vi "Field Draw Robot.vi"(0 "Offset":T5, 1 "picture in":picture, 3 "Draw Number":bool, 5 "Robot":refnum<class "Robot.lvclass">=refnum, 6 "Project":T1=enum."VSS", 7 "Game in":refnum<class "Game.lvclass">=refnum, 9 "Scale mm/pixel":sgl, 11 "color(black)":u32(colorbox)=16775978, 12 "Lado":enum16{"Esquerdo", "Direito"}(ring), 14 "color":enum16{"Azul", "Amarelo"}(ring), 15 "Draw Targets?":T3) -> (4 "picture out":picture)   [LabVIEW 2022 SP3]
uses:
  <vilib>/Analysis/NI_AALPro.lvlib
  <vilib>/Analysis/coordinate.llb/2D Cartesian Coordinate Rotation (Scalar).vi
  Controls/Functions Enum.ctl
  Robot_class/Robot.lvclass
  Game_class/Game.lvclass
  Enemy_class/Enemy.lvclass
  Referee_class/Referee.lvclass
  <vilib>/Utility/miscctls.llb/LVBoundsTypeDef.ctl
  DrawTargets.ctl
  Project.ctl
panel:
  in  "pen Chute 2":T2={"Width"=3, "Style"=enum."Solid"}
  in  "pen Chute":T2={"Width"=3, "Style"=enum."Solid"}
  in  "pen":T4={"Width"=1.0, "Style"=enum."Solid"}
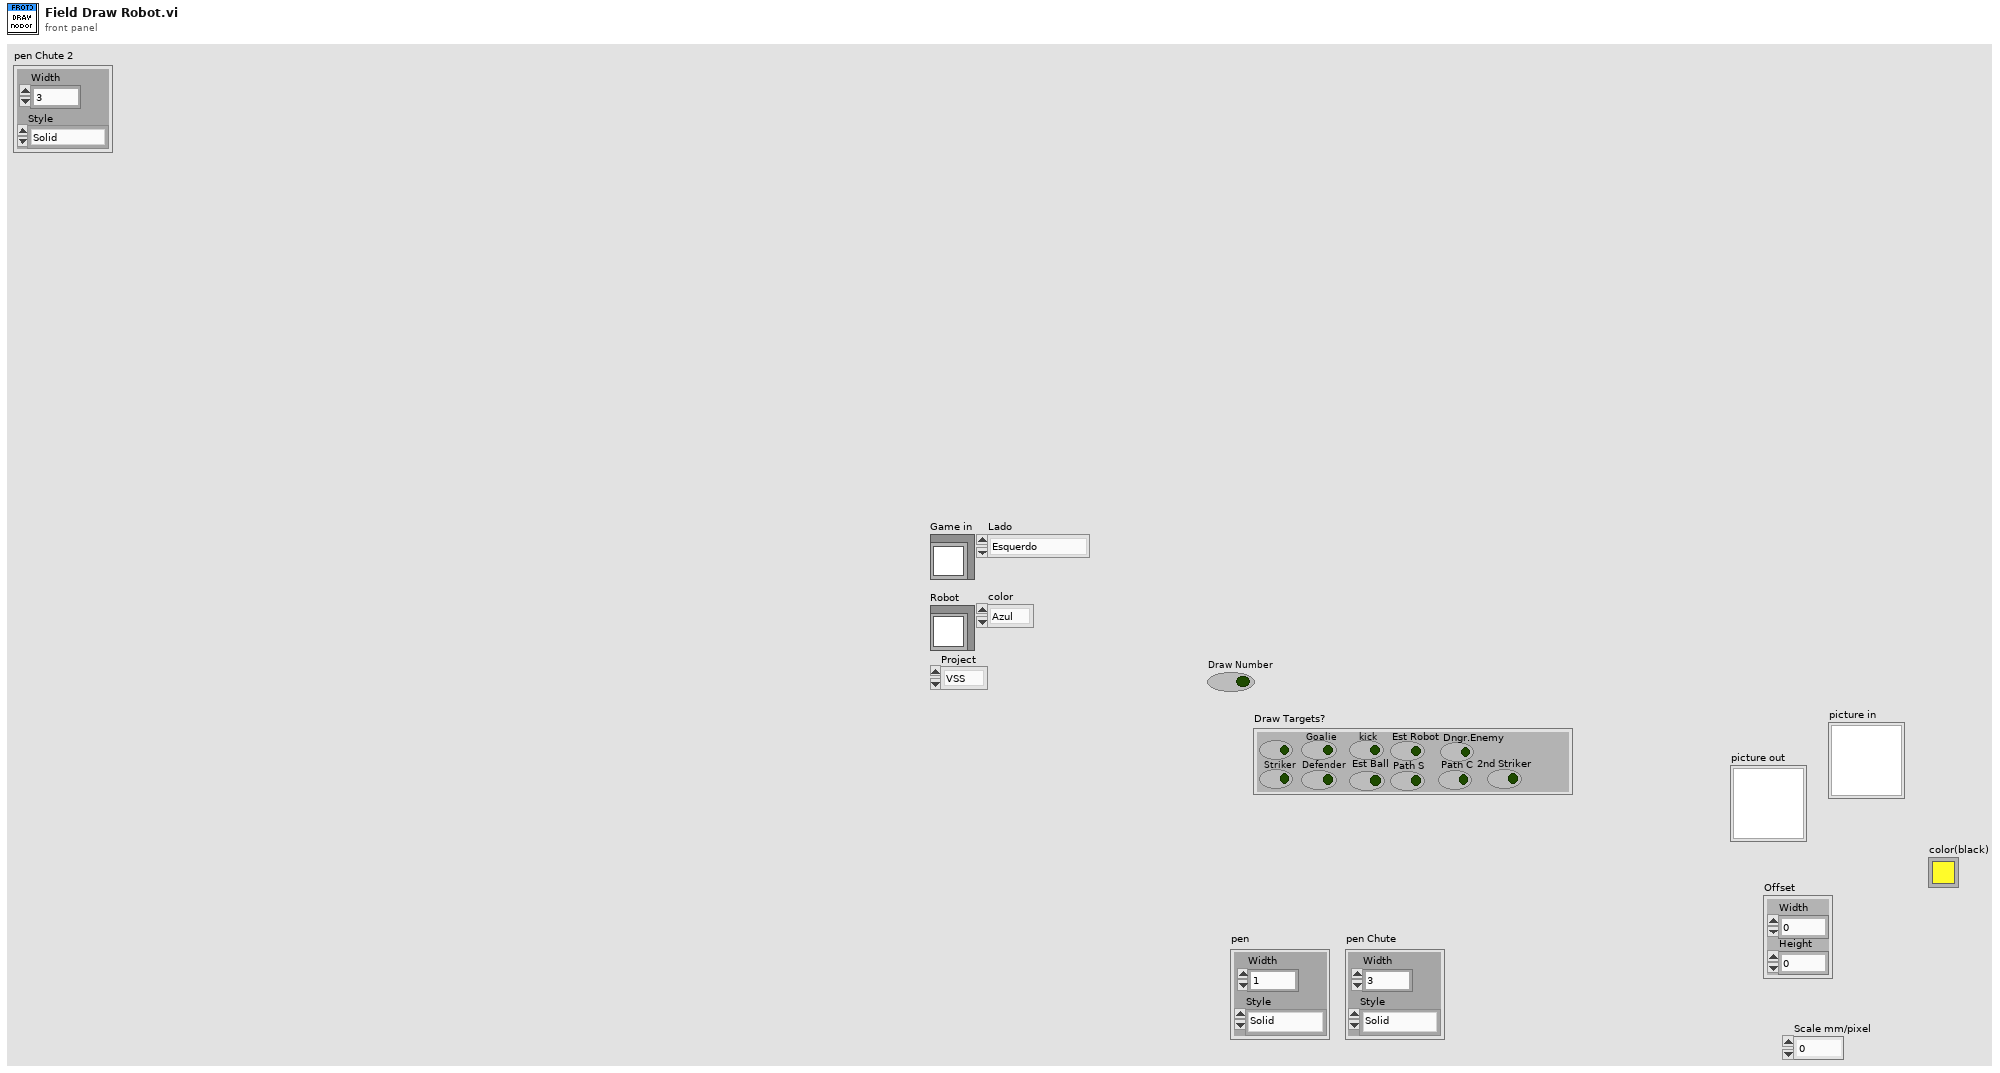
[diagram p1: front panel]
types:
  T1 = typedef "Project.ctl" = enum16{"SSL", "VSS"}
  T2 = cluster{"Width":u16, "Style":enum32{"Solid", "Dash", "Dot", "DashDot", "DashDotDot"}}
  T3 = typedef "DrawTargets.ctl" = cluster{"Attacker":bool, "Striker":bool, "Goalie":bool, "Defender":bool, "kick":bool, "Est Ball":bool, "Est Robot":bool, "Path S":bool, "Path C":bool, "Dngr.Enemy":bool, "2nd Striker":bool}
  T4 = cluster{"Width":dbl, "Style":enum32{"Solid", "Dash", "Dot", "DashDot", "DashDotDot"}}
  T5 = typedef "LVBoundsTypeDef.ctl" = cluster{"Width":u32, "Height":u32}
  T6 = typedef "Functions Enum.ctl" = enum16{"2nd Striker", "Attacker", "Goalie", "Defender", "Striker", "Goto 0", "Dummy", "Kicker", "ZigZag 0", "ZigZag 1", "ZigZag 2", "ZigZag 3", "ZigZag 4", "ZigZag 5", "ZigZag 6", "ZigZag 7", "ZigZag 8", ""}
  T7 = cluster{"horizontal":enum16{"left", "center", "right"}, "vertical":enum16{"top", "center", "bottom"}}
  T8 = typedef "dangerEnemy.ctl" = cluster{"dangerFactor":dbl, "allyRobotId":i32, "enemyRobotId":i32}
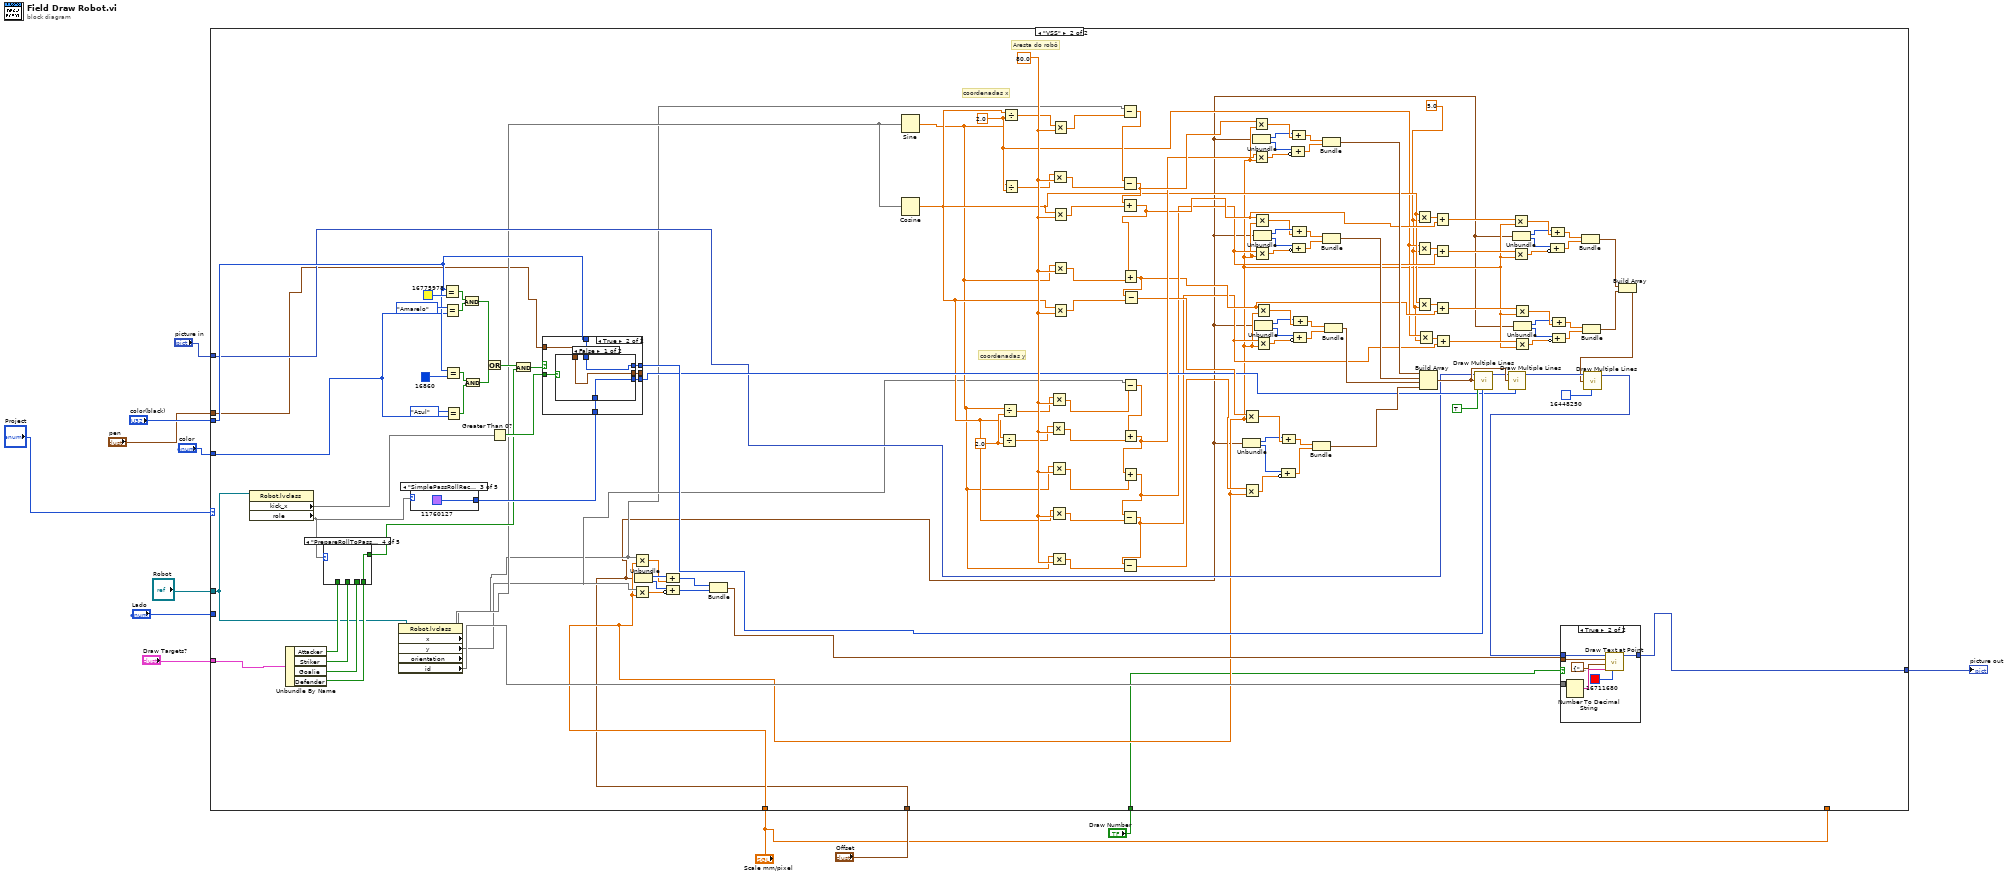
[diagram p0: block diagram]
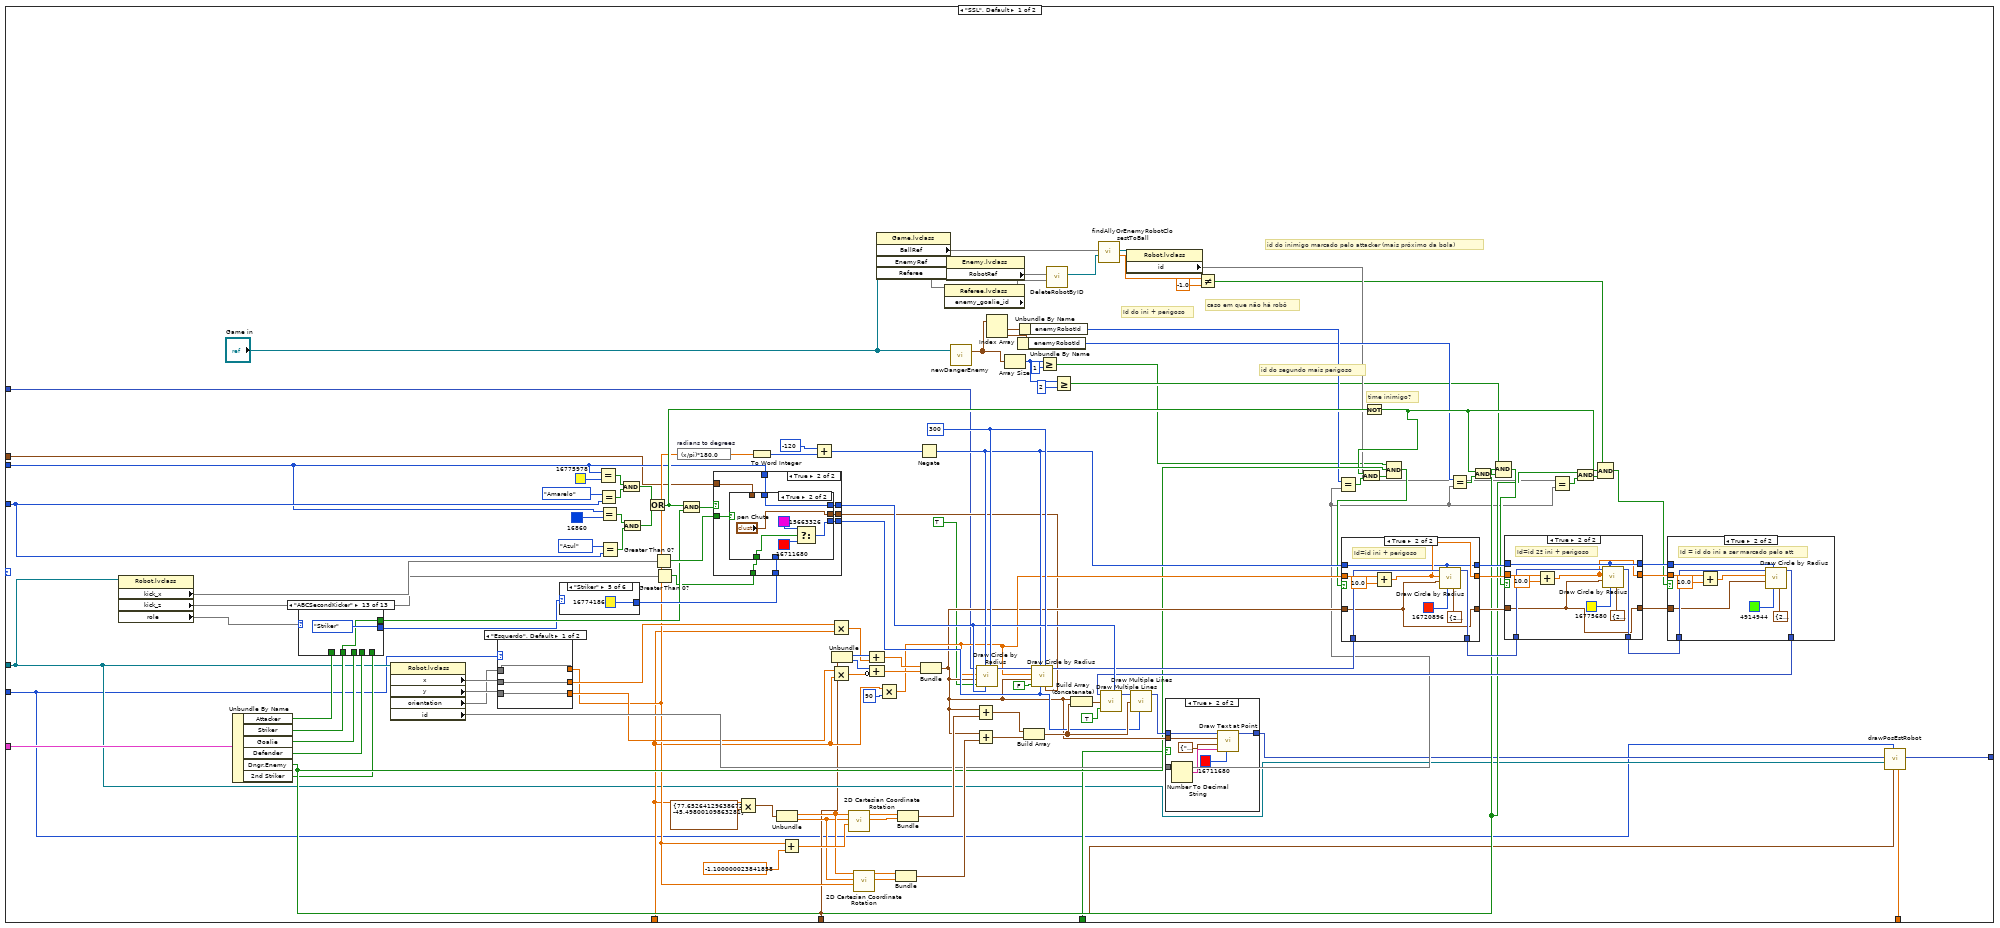
[diagram p2: hidden frame]
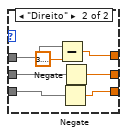
[diagram p3: hidden frame]
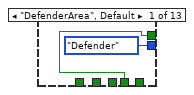
[diagram p7: hidden frame]
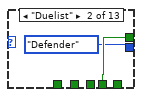
[diagram p8: hidden frame]
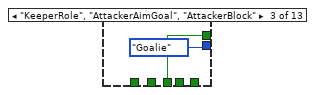
[diagram p9: hidden frame]
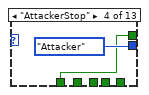
[diagram p10: hidden frame]
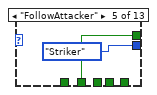
[diagram p11: hidden frame]
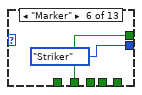
[diagram p12: hidden frame]
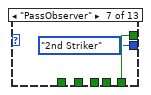
[diagram p13: hidden frame]
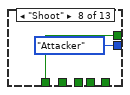
[diagram p14: hidden frame]
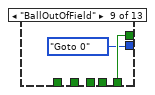
[diagram p15: hidden frame]
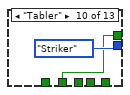
[diagram p16: hidden frame]
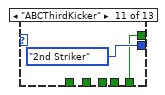
[diagram p17: hidden frame]
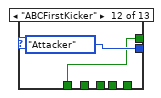
[diagram p18: hidden frame]
diagram:
  n1 = case shown="\"VSS\"" "Project" {
    tunnel: "Robot" -> [w19 w252]
    tunnel: "Draw Targets?" -> [w49 w257]
    tunnel: "color" -> [w48 w246]
    tunnel: "color(black)" -> [w47 w261]
    tunnel: [w17 w247] -> w8
    tunnel: "Draw Number" -> [w46 w248]
    tunnel: "picture in" -> [w45 w258]
    tunnel: "pen" -> [w44 w251]
    tunnel: "Offset" -> [w18 w249]
    tunnel: "Scale mm/pixel" -> [w43 w250]
    tunnel: "Lado" -> [w15 _]
    tunnel: "Scale mm/pixel" -> [w16 _]
    frame "SSL", Default {
      w129 = i16 300 ("arc size(360)")
      # "caso em que não há robô"
      # "id do inimigo marcado pelo attacker (mais próximo da bola)"
      # "id do segundo mais perigoso"
      # "time inimigo?"
      # "Id do ini + perigoso"
      n2 = property class="Robot.lvclass"(reference=w19) -> ("kick_x"=w58, "kick_z"=w14, "role"=w56)  [unwired: 1 in, 2 out]
      n3 = Unbundle By Name(w49) -> ("Attacker"=w93:bool, "Striker"=w92:bool, "Goalie"=w91:bool, "Defender"=w90:bool, "Dngr.Enemy"=w63:bool, "2nd Striker"=w60:bool)
      n4 = case shown="\"ABCSecondKicker\"" w56 {
        tunnel: [w187 w190 w192 w193 w196 w198 w200 w202 w204 w205 w207 w209 w211] -> w88
        tunnel: w90 -> [w187 w190 _ _ _ _ _ _ _ _ _ _ _]
        tunnel: w92 -> [_ _ _ _ w196 w198 _ _ _ w205 _ _ w211]
        tunnel: w93 -> [_ _ _ w193 _ _ _ w202 _ _ _ w209 _]
        tunnel: w91 -> [_ _ w192 _ _ _ _ _ _ _ _ _ _]
        tunnel: w60 -> [_ _ _ _ _ _ w200 _ w204 _ w207 _ _]
        tunnel: [Functions_Enum."Defender" ("function") Functions_Enum."Defender" ("function") Functions_Enum."Goalie" ("function") Functions_Enum."Attacker" ("function") Functions_Enum."Striker" ("function") Functions_Enum."Striker" ("function") Functions_Enum."2nd Striker" ("function") Functions_Enum."Attacker" ("function") Functions_Enum."Goto 0" ("function") Functions_Enum."Striker" ("function") Functions_Enum."2nd Striker" ("function") Functions_Enum."Attacker" ("function") Functions_Enum."Striker" ("function")] -> w57
        frame "DefenderArea", Default {
        }
        frame "Duelist" {
        }
        frame "KeeperRole", "AttackerAimGoal", "AttackerBlock" {
        }
        frame "AttackerStop" {
        }
        frame "FollowAttacker" {
        }
        frame "Marker" {
        }
        frame "PassObserver" {
        }
        frame "Shoot" {
        }
        frame "BallOutOfField" {
        }
        frame "Tabler" {
        }
        frame "ABCThirdKicker" {
        }
        frame "ABCFirstKicker" {
        }
        frame "ABCSecondKicker" {
        }
      }
      n5 = property class="Robot.lvclass"(reference=w19) -> ("x"=w55, "y"=w53, "orientation"=w51, "id"=w59)  [unwired: 1 in, 2 out]
      n6 = case shown="\"Esquerdo\", Default" w15 {
        tunnel: [w143 w150] -> w54
        tunnel: w55 -> [w143 w147]
        tunnel: [w142 w148] -> w52
        tunnel: w53 -> [w142 w149]
        tunnel: w51 -> [w141 w145]
        tunnel: [w141 w146] -> w50
        frame "Esquerdo", Default {
        }
        frame "Direito" {
          n7 = Subtract(x=w145, y=3.141592653589793) -> (x-y=w146:dbl)
          n8 = Negate(x=w149) -> (-x=w148:dbl)
          n9 = Negate(x=w147) -> (-x=w150:dbl)
        }
      }
      n10 = case shown="\"Striker\"" w57 {
        tunnel: [u32 14047743 ("color(black)") u32 16711680 ("color(black)") u32 11760127 ("color(black)") u32 4390883 ("color(black)") u32 16774186 ("color(black)") u32 197379 ("color(black)")] -> w95
        frame "Goalie" {
        }
        frame "Attacker", Default {
        }
        frame "Goto 0", "Kicker", "ZigZag 0" {
        }
        frame "Defender" {
        }
        frame "Striker" {
        }
        frame "2nd Striker" {
        }
      }
      n11 = Equal?(x=w47, y=u32 16775978 ("color(black)")) -> (x = y?=w102:bool)
      n12 = Equal?(x=enum16{"Azul", "Amarelo"}."Amarelo", y=w48) -> (x = y?=w103:bool)
      n13 = Equal?(x=w47, y=u32 16860 ("color(black)")) -> (x = y?=w99:bool)
      n14 = Equal?(x=enum16{"Azul", "Amarelo"}."Azul", y=w48) -> (x = y?=w100:bool)
      n15 = And(x=w102, y=w103) -> (x .and. y?=w97:bool)
      n16 = And(x=w99, y=w100) -> (x .and. y?=w96:bool)
      n17 = Or(x=w97, y=w96) -> (x .or. y?=w74:bool)
      n18 = Greater Than 0?(x=w58) -> (x > 0?=w94:bool)
      n19 = Greater Than 0?(x=w14) -> (x > 0?=w13:bool)
      n20 = expression code="(x/pi)*180.0" "radians to degrees"(w50) -> (w132:dbl)
      n21 = And(x=w74, y=w88) -> (x .and. y?=w89:bool)
      n22 = case shown="True" w89 {
        tunnel: [w214 w222] -> w107
        tunnel: [w214 w221] -> w106
        tunnel: w47 -> [w214 w220]
        tunnel: w95 -> [_ w219]
        tunnel: [w213 w218] -> w82
        tunnel: w94 -> [_ w217]
        tunnel: w44 -> [w213 w216]
        tunnel: w13 -> [_ w215]
        frame False {
        }
        frame True {
          n23 = case shown="True" w217 {
            tunnel: [w224 w226] -> w221
            tunnel: w220 -> [w225 w231]
            tunnel: [w225 w231] -> w222
            tunnel: w219 -> [w224 _]
            tunnel: [w223 "pen Chute"] -> w218
            tunnel: w216 -> [w223 _]
            tunnel: w215 -> [_ w229]
            frame False {
            }
            frame True {
              n24 = Select(t=u32 15663326 ("color(black)"), s=w229, f=u32 16711680 ("color(black)")) -> (s? t:f=w226:u32)
            }
          }
        }
      }
      n25 = Multiply(x=w43, y=cluster{sgl, sgl} {77.65264, -45.498} ("appended array")) -> (x*y=w113:cluster{sgl, sgl})
      n26 = To Word Integer(number=w132) -> (16bit integer=w131:i16)
      n27 = Unbundle(w113) -> (w118:sgl, w117:sgl)
      n28 = Add(x=w50, y=sgl -1.1 ("theta")) -> (x+y=w119:sgl)
      n29 = Add(x=i16 -120, y=w131) -> (x+y=w130:i16)
      n30 = Multiply(x=w54, y=w43) -> (x*y=w138:sgl)
      n31 = Multiply(x=w52, y=w43) -> (x*y=w135:sgl)
      n32 = Unbundle(w18) -> ("Width"=w139:u32, "Height"=w136:u32)
      n33 = call-poly <vilib>:"2D Cartesian Coordinate Rotation.vi"("theta"=w119, "y"=w117, "x"=w118) -> ("y out"=w121:dbl, "x out"=w122:dbl)  [unwired: 6 in, 1 out]
      n34 = call-poly <vilib>:"2D Cartesian Coordinate Rotation.vi"("theta"=w50, "y"=w117, "x"=w118) -> ("y out"=w115:dbl, "x out"=w116:dbl)  [unwired: 6 in, 1 out]
      n35 = Compound Arithmetic op=ADD(w139, w138) -> (w137:sgl)
      n36 = Compound Arithmetic op=ADD(w136, invert w135) -> (w134:sgl)
      n37 = property class="Game.lvclass"(reference="Game in") -> ("BallRef"=w36, "EnemyRef"=w35, "Referee"=w30)  [unwired: 1 in, 2 out]
      n38 = Multiply(x=w43, y=i16 90 ("radius")) -> (x*y=w85:sgl)
      n39 = Bundle("x out"=w116, "y out"=w115) -> (w112:cluster{"x out":dbl, "y out":dbl})  [unwired: 1 in]
      n40 = Bundle("x out"=w122, "y out"=w121) -> (w111:cluster{"x out":dbl, "y out":dbl})  [unwired: 1 in]
      n41 = Negate(x=w130) -> (-x=w87:i16)
      n42 = Bundle(w137, w134) -> (w84:cluster{sgl, sgl})  [unwired: 1 in]
      n43 = property class="Referee.lvclass"(reference=w30) -> ("enemy_goalie_id"=w24)  [unwired: 1 in, 2 out]
      n44 = property class="Enemy.lvclass"(reference=w35) -> ("RobotRef"=w25)  [unwired: 1 in, 2 out]
      n45 = call "newDangerEnemy.vi"("Game"="Game in") -> ("dangerEnemies"=w34:T8[])  [unwired: 11 in, 3 out]
      n46 = Add(x=w84, y=w111) -> (x+y=w109:cluster{dbl, dbl})
      n47 = Add(x=w84, y=w112) -> (x+y=w110:cluster{sgl, sgl})
      n48 = call <vilib>:"Draw Circle by Radius.vi"("arc size(360)"=w129, "color(black)"=w107, "start angle(0)"=w87, "fill?(F)"=TRUE, "pixel center"=w84, "radius"=w85, "picture"=w45) -> ("new picture"=w108:picture)  [unwired: 4 in]
      n49 = Index Array(array=w34) -> (element #1=w42:T8, element #2=w40:T8)  [unwired: 2 in]
      n50 = Array Size(array=w34) -> (size(s)=w31:i32)
      n51 = Unbundle By Name(w40) -> ("enemyRobotId"=w39:i32)
      n52 = Unbundle By Name(w42) -> ("enemyRobotId"=w41:i32)
      n53 = Build Array(w109, w110) -> (w126:cluster{dbl, dbl}[])
      n54 = call <vilib>:"Draw Circle by Radius.vi"("pen"=w82, "arc size(360)"=w129, "color(black)"=w106, "start angle(0)"=w87, "fill?(F)"=FALSE, "pixel center"=w84, "radius"=w85, "picture"=w108) -> ("new picture"=w86:picture)  [unwired: 3 in]
      n55 = Greater Or Equal?(x=w31, y=1) -> (x >= y?=w26:bool)
      n56 = call "DeleteRobotByID.vi"("id"=w24, "RobotRef"=w25) -> ("RobotRef out"=w23:refnum<class "Robot.lvclass">[])  [unwired: 7 in, 2 out]
      n57 = Greater Or Equal?(x=w31, y=2) -> (x >= y?=w27:bool)
      n58 = Build Array (concatenate)(w84, w126) -> (w124:cluster{dbl, dbl}[])
      n59 = call "findAllyOrEnemyRobotClosestToBall.vi"("Ally/Enemy Robots"=w23, "Ball"=w36) -> ("Robot distance to ball"=w22:dbl, "Robot"=w38:refnum<class "Robot.lvclass">)  [unwired: 6 in, 2 out]
      n60 = property class="Robot.lvclass"(reference=w38) -> ("id"=w29)  [unwired: 1 in, 2 out]
      n61 = Not Equal?(x=w22, y=-1.0) -> (x != y?=w28:bool)
      n62 = Equal?(x=w41, y=w59) -> (x = y?=w81:bool)
      n63 = Not(x=w74) -> (.not. x?=w62:bool)
      n64 = And(x=w62, y=w81) -> (x .and. y?=w75:bool)
      n65 = Compound Arithmetic op=AND(w26, w63, w75) -> (w73:bool)
      n66 = case shown="True" w73 {
        tunnel: w87 -> [w176 w179]
        tunnel: w86 -> [w177 w186]
        tunnel: [w177 w185] -> w79
        tunnel: w85 -> [w175 w184]
        tunnel: w84 -> [w174 w178]
        tunnel: [w176 w179] -> w78
        tunnel: [w175 w180] -> w77
        tunnel: [w174 w178] -> w76
        frame False {
        }
        frame True {
          # "Id=id ini + perigoso"
          n67 = Add(x=w184, y=sgl 10.0) -> (x+y=w180:sgl)
          n68 = call <vilib>:"Draw Circle by Radius.vi"("pen"=T2 {"Width"=2, "Style"=enum."Solid"}, "color(black)"=u32 16720896, "start angle(0)"=w179, "pixel center"=w178, "radius"=w180, "picture"=w186) -> ("new picture"=w185:picture)  [unwired: 5 in]
        }
      }
      n69 = Equal?(x=w39, y=w59) -> (x = y?=w80:bool)
      n70 = And(x=w62, y=w80) -> (x .and. y?=w72:bool)
      n71 = Compound Arithmetic op=AND(w27, w63, w72) -> (w71:bool)
      n72 = case shown="True" w71 {
        tunnel: w78 -> [w163 w167]
        tunnel: w79 -> [w164 w173]
        tunnel: [w164 w172] -> w67
        tunnel: w77 -> [w162 w171]
        tunnel: w76 -> [w161 w165]
        tunnel: [w163 w167] -> w70
        tunnel: [w162 w166] -> w69
        tunnel: [w161 w165] -> w68
        frame False {
        }
        frame True {
          # "Id=id 2º ini + perigoso"
          n73 = Add(x=w171, y=sgl 10.0) -> (x+y=w166:sgl)
          n74 = call <vilib>:"Draw Circle by Radius.vi"("pen"=T2 {"Width"=2, "Style"=enum."Solid"}, "color(black)"=u32 16775680, "start angle(0)"=w167, "pixel center"=w165, "radius"=w166, "picture"=w173) -> ("new picture"=w172:picture)  [unwired: 5 in]
        }
      }
      n75 = Equal?(x=w29, y=w59) -> (x = y?=w64:bool)
      n76 = And(x=w63, y=w64) -> (x .and. y?=w65:bool)
      n77 = Compound Arithmetic op=AND(w28, w62, w65) -> (w61:bool)
      n78 = case shown="True" w61 {
        tunnel: w70 -> [_ w160]
        tunnel: w67 -> [w151 w159]
        tunnel: [w151 w158] -> w66
        tunnel: w69 -> [_ w157]
        tunnel: w68 -> [_ w156]
        frame False {
        }
        frame True {
          # "Id = id do ini a ser marcado pelo att"
          n79 = Add(x=w157, y=sgl 10.0) -> (x+y=w155:sgl)
          n80 = call <vilib>:"Draw Circle by Radius.vi"("pen"=T2 {"Width"=2, "Style"=enum."Solid"}, "color(black)"=u32 4914944, "start angle(0)"=w160, "pixel center"=w156, "radius"=w155, "picture"=w159) -> ("new picture"=w158:picture)  [unwired: 5 in]
        }
      }
      n81 = call <vilib>:"Draw Multiple Lines.vi"("picture"=w66, "line endpoints"=w124, "fill?(F)"=TRUE, "color(black)"=w107) -> ("new picture"=w125:picture)  [unwired: 5 in]
      n82 = call <vilib>:"Draw Multiple Lines.vi"("picture"=w125, "line endpoints"=w126, "color(black)"=w106) -> ("new picture"=w127:picture)  [unwired: 6 in]
      n83 = case shown="True" w46 {
        tunnel: [w238 w245] -> w20
        tunnel: w59 -> [_ w243]
        tunnel: w127 -> [w238 w241]
        tunnel: w84 -> [_ w240]
        frame False {
        }
        frame True {
          n84 = Number To Decimal String(number=w243) -> (decimal integer string=w244:string)  [unwired: 1 in]
          n85 = call <vilib>:"Draw Text at Point.vi"("text color(black)"=u32 16711680, "text"=w244, "alignment(left, top)"=T7 {"horizontal"=enum."center", "vertical"=enum."center"}, "origin"=w240, "picture"=w241) -> ("new picture"=w245:picture)  [unwired: 5 in, 1 out]
        }
      }
      n86 = call "drawPosEstRobot.vi"("Scale"=w16, "Offset"=w18, "Lado"=w15, "Robot"=w19, "Picture In"=w20) -> ("picture out"=w17:picture)  [unwired: 4 in, 2 out]
    }
    frame "VSS" {
      w268 = 5.0 ("y")
      w313 = 80.0 ("y")
      w348 = 2.0 ("y")
      w350 = 2.0 ("y")
      # "coordenadas y"
      # "Aresta do robô"
      # "coordenadas x"
      n87 = property class="Robot.lvclass"(reference=w252) -> ("kick_x"=w260, "role"=w259)  [unwired: 1 in, 2 out]
      n88 = Unbundle By Name(w257) -> ("Attacker"=w357:bool, "Striker"=w356:bool, "Goalie"=w355:bool, "Defender"=w354:bool)
      n89 = case shown="\"PrepareRollToPassReceiver\"" w259 {
        tunnel: [w377 w378 TRUE ("Draw Target Striker?") w380 w381] -> w351
        tunnel: w354 -> [_ _ _ w380 _]
        tunnel: w356 -> [_ _ _ _ w381]
        tunnel: w357 -> [w377 _ _ _ _]
        tunnel: w355 -> [_ w378 _ _ _]
        frame "TableFinalizer", Default {
        }
        frame "PrepareRollToPassRoller" {
        }
        frame "SimplePassRollReceiver", "PreparePassReceiver 2" {
        }
        frame "PrepareRollToPassReceiver" {
        }
        frame "SimplePassRoll" {
        }
      }
      n90 = property class="Robot.lvclass"(reference=w252) -> ("x"=w253, "y"=w254, "orientation"=w255, "id"=w256)  [unwired: 1 in, 2 out]
      n91 = case shown="\"SimplePassRollReceiver\", \"PreparePassReceiver 2\"" w259 {
        tunnel: [u32 14047743 ("color(black)") u32 16711686 ("color(black)") u32 11760127 ("color(black)") u32 4390883 ("color(black)") u32 16774186 ("color(black)")] -> w359
        frame "PrepareRollToPassRoller" {
        }
        frame "TableFinalizer", Default {
        }
        frame "SimplePassRollReceiver", "PreparePassReceiver 2" {
        }
        frame "PrepareRollToPassReceiver" {
        }
        frame "SimplePassRoll" {
        }
      }
      n92 = Equal?(x=w261, y=u32 16775978 ("color(black)")) -> (x = y?=w366:bool)
      n93 = Equal?(x=enum16{"Azul", "Amarelo"}."Amarelo", y=w246) -> (x = y?=w367:bool)
      n94 = Equal?(x=w261, y=u32 16860 ("color(black)")) -> (x = y?=w363:bool)
      n95 = Equal?(x=enum16{"Azul", "Amarelo"}."Azul", y=w246) -> (x = y?=w364:bool)
      n96 = And(x=w366, y=w367) -> (x .and. y?=w361:bool)
      n97 = And(x=w363, y=w364) -> (x .and. y?=w360:bool)
      n98 = Or(x=w361, y=w360) -> (x .or. y?=w352:bool)
      n99 = Greater Than 0?(x=w260) -> (x > 0?=w358:bool)
      n100 = And(x=w352, y=w351) -> (x .and. y?=w353:bool)
      n101 = case shown="True" w353 {
        tunnel: [w383 w390] -> w298
        tunnel: [w383 w389] -> w295
        tunnel: w261 -> [w383 w388]
        tunnel: w359 -> [_ w387]
        tunnel: [w382 w386] -> _
        tunnel: w358 -> [_ w385]
        tunnel: w251 -> [w382 w384]
        frame False {
        }
        frame True {
          n102 = case shown="False" w385 {
            tunnel: [w392 u32 16711680 ("color(black)")] -> w389
            tunnel: w388 -> [w393 w395]
            tunnel: [w393 w395] -> w390
            tunnel: w387 -> [w392 _]
            tunnel: [w391 "pen Chute 2"] -> w386
            tunnel: w384 -> [w391 _]
            frame False {
            }
            frame True {
            }
          }
        }
      }
      n103 = Multiply(x=w253, y=w250) -> (x*y=w375:sgl)
      n104 = Multiply(x=w254, y=w250) -> (x*y=w372:sgl)
      n105 = Unbundle(w249) -> ("Width"=w376:u32, "Height"=w373:u32)
      n106 = Compound Arithmetic op=ADD(w376, w375) -> (w374:u32)
      n107 = Compound Arithmetic op=ADD(w373, invert w372) -> (w371:u32)
      n108 = Bundle(w374, w371) -> (w370:cluster{u32, u32})  [unwired: 1 in]
      n109 = Sine(x=w255) -> (sin(x)=w269:dbl)
      n110 = Cosine(x=w255) -> (cos(x)=w270:dbl)
      n111 = Divide(x=w270, y=w348) -> (x/y=w303:dbl)
      n112 = Divide(x=w269, y=w348) -> (x/y=w305:dbl)
      n113 = Divide(x=w270, y=w350) -> (x/y=w312:dbl)
      n114 = Divide(x=w269, y=w350) -> (x/y=w310:dbl)
      n115 = Multiply(x=w303, y=w313) -> (x*y=w302:dbl)
      n116 = Multiply(x=w305, y=w313) -> (x*y=w304:dbl)
      n117 = Multiply(x=w269, y=w313) -> (x*y=w301:dbl)
      n118 = Multiply(x=w270, y=w313) -> (x*y=w300:dbl)
      n119 = Multiply(x=w269, y=w313) -> (x*y=w299:dbl)
      n120 = Multiply(x=w310, y=w313) -> (x*y=w309:dbl)
      n121 = Multiply(x=w312, y=w313) -> (x*y=w311:dbl)
      n122 = Multiply(x=w270, y=w313) -> (x*y=w308:dbl)
      n123 = Multiply(x=w269, y=w313) -> (x*y=w307:dbl)
      n124 = Multiply(x=w270, y=w313) -> (x*y=w306:dbl)
      n125 = Subtract(x=w253, y=w311) -> (x-y=w349:dbl)
      n126 = Subtract(x=w349, y=w309) -> (x-y=w335:dbl)
      n127 = Add(x=w335, y=w308) -> (x+y=w274:dbl)
      n128 = Add(x=w274, y=w307) -> (x+y=w272:dbl)
      n129 = Subtract(x=w254, y=w304) -> (x-y=w347:dbl)
      n130 = Add(x=w347, y=w302) -> (x+y=w334:dbl)
      n131 = Add(x=w334, y=w301) -> (x+y=w273:dbl)
      n132 = Subtract(x=w273, y=w300) -> (x-y=w271:dbl)
      n133 = Subtract(x=w271, y=w299) -> (x-y=w316:dbl)
      n134 = Subtract(x=w272, y=w306) -> (x-y=w317:dbl)
      n135 = Multiply(x=w317, y=w250) -> (x*y=w345:dbl)
      n136 = Unbundle(w249) -> ("Width"=w344:u32, "Height"=w342:u32)
      n137 = Multiply(x=w316, y=w250) -> (x*y=w343:dbl)
      n138 = Multiply(x=w335, y=w250) -> (x*y=w336:dbl)
      n139 = Unbundle(w249) -> ("Width"=w333:u32, "Height"=w332:u32)
      n140 = Multiply(x=w334, y=w250) -> (x*y=w337:dbl)
      n141 = Multiply(x=w274, y=w250) -> (x*y=w328:dbl)
      n142 = Unbundle(w249) -> ("Width"=w329:u32, "Height"=w330:u32)
      n143 = Multiply(x=w273, y=w250) -> (x*y=w327:dbl)
      n144 = Multiply(x=w272, y=w250) -> (x*y=w320:dbl)
      n145 = Unbundle(w249) -> ("Width"=w319:u32, "Height"=w318:u32)
      n146 = Multiply(x=w271, y=w250) -> (x*y=w321:dbl)
      n147 = Compound Arithmetic op=ADD(w342, invert w343) -> (w341:dbl)
      n148 = Compound Arithmetic op=ADD(w344, w345) -> (w340:dbl)
      n149 = Compound Arithmetic op=ADD(w332, invert w337) -> (w338:dbl)
      n150 = Compound Arithmetic op=ADD(w333, w336) -> (w339:dbl)
      n151 = Compound Arithmetic op=ADD(w330, invert w327) -> (w326:dbl)
      n152 = Compound Arithmetic op=ADD(w329, w328) -> (w325:dbl)
      n153 = Compound Arithmetic op=ADD(w318, invert w321) -> (w322:dbl)
      n154 = Compound Arithmetic op=ADD(w319, w320) -> (w323:dbl)
      n155 = Bundle(w340, w341) -> (w315:cluster{dbl, dbl})  [unwired: 1 in]
      n156 = Bundle(w339, w338) -> (w331:cluster{dbl, dbl})  [unwired: 1 in]
      n157 = Bundle(w325, w326) -> (w324:cluster{dbl, dbl})  [unwired: 1 in]
      n158 = Bundle(w323, w322) -> (w314:cluster{dbl, dbl})  [unwired: 1 in]
      n159 = Multiply(x=w270, y=w268) -> (x*y=w278:dbl)
      n160 = Multiply(x=w269, y=w268) -> (x*y=w277:dbl)
      n161 = Multiply(x=w270, y=w268) -> (x*y=w276:dbl)
      n162 = Multiply(x=w269, y=w268) -> (x*y=w275:dbl)
      n163 = Build Array(w331, w324, w314, w315) -> (w297:cluster{dbl, dbl}[])
      n164 = Add(x=w278, y=w274) -> (x+y=w282:dbl)
      n165 = Add(x=w277, y=w273) -> (x+y=w281:dbl)
      n166 = Add(x=w276, y=w272) -> (x+y=w280:dbl)
      n167 = Add(x=w275, y=w271) -> (x+y=w279:dbl)
      n168 = call <vilib>:"Draw Multiple Lines.vi"("picture"=w258, "line endpoints"=w297, "fill?(F)"=TRUE, "color(black)"=w298) -> ("new picture"=w296:picture)  [unwired: 5 in]
      n169 = call <vilib>:"Draw Multiple Lines.vi"("picture"=w296, "line endpoints"=w297, "color(black)"=w295) -> ("new picture"=w267:picture)  [unwired: 6 in]
      n170 = Multiply(x=w282, y=w250) -> (x*y=w287:dbl)
      n171 = Unbundle(w249) -> ("Width"=w286:u32, "Height"=w285:u32)
      n172 = Multiply(x=w281, y=w250) -> (x*y=w288:dbl)
      n173 = Multiply(x=w280, y=w250) -> (x*y=w294:dbl)
      n174 = Unbundle(w249) -> ("Width"=w284:u32, "Height"=w283:u32)
      n175 = Multiply(x=w279, y=w250) -> (x*y=w293:dbl)
      n176 = Compound Arithmetic op=ADD(w285, invert w288) -> (w289:dbl)
      n177 = Compound Arithmetic op=ADD(w286, w287) -> (w290:dbl)
      n178 = Compound Arithmetic op=ADD(w283, invert w293) -> (w292:dbl)
      n179 = Compound Arithmetic op=ADD(w284, w294) -> (w291:dbl)
      n180 = Bundle(w290, w289) -> (w265:cluster{dbl, dbl})  [unwired: 1 in]
      n181 = Bundle(w291, w292) -> (w264:cluster{dbl, dbl})  [unwired: 1 in]
      n182 = Build Array(w265, w264) -> (w263:cluster{dbl, dbl}[])
      n183 = call <vilib>:"Draw Multiple Lines.vi"("picture"=w267, "line endpoints"=w263, "color(black)"=u32 16448250) -> ("new picture"=w266:picture)  [unwired: 6 in]
      n184 = case shown="True" w248 {
        tunnel: [w402 w409] -> w247
        tunnel: w256 -> [_ w407]
        tunnel: w266 -> [w402 w405]
        tunnel: w370 -> [_ w404]
        frame False {
        }
        frame True {
          n185 = Number To Decimal String(number=w407) -> (decimal integer string=w408:string)  [unwired: 1 in]
          n186 = call <vilib>:"Draw Text at Point.vi"("text color(black)"=u32 16711680, "text"=w408, "alignment(left, top)"=T7 {"horizontal"=enum."center", "vertical"=enum."center"}, "origin"=w404, "picture"=w405) -> ("new picture"=w409:picture)  [unwired: 5 in, 1 out]
        }
      }
    }
  }
  "picture out" <- w8
